vi "JSON Tree to MuxList.vi"(8 "error in (no error)":errorcluster, 11 "JSON Array":variant) -> (0 "error out":errorcluster, 2 "MuxList":cluster{"Src":string, "Dests":string[]}[](array[cluster]), 3 "JSON Tree Passthrough (JSON Array)":variant)   [LabVIEW 2015, in "SLSC Switch.lvlib" / "SLSC Switch.lvclass"]
uses:
  SLSC Switch.lvclass
  <vilib>/LVH/i3 JSON/JSON Parsing/Get Object Parameter Files/Get Object Parameter - Array.vi
  <vilib>/LVH/i3 JSON/JSON Parsing/Get Array Value at Index Files/Get Array Value at Index - Object.vi
  <vilib>/LVH/i3 JSON/JSON Parsing/Get Object Parameter Files/Get Object Parameter - String.vi
  <vilib>/LVH/i3 JSON/i3-json.lvlib
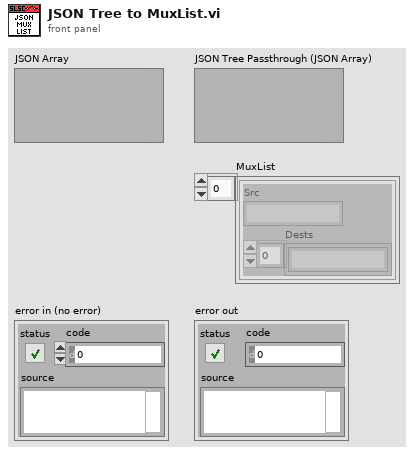
[diagram p1: front panel]
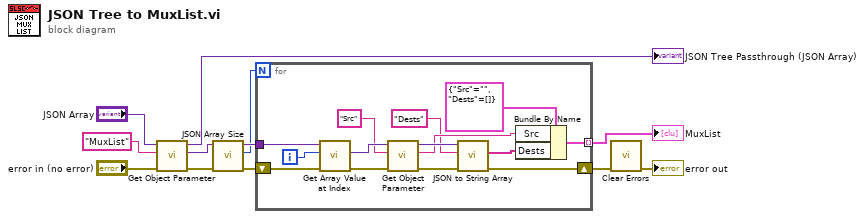
[diagram p0: block diagram]
diagram:
  n1 = call-poly <vilib>:"Get Object Parameter.vi"("error in (no error)"="error in (no error)", "Parameter Name"="MuxList", "JSON Tree In (JSON Object)"="JSON Array") -> ("error out"=w6:errorcluster, "JSON Array"=w5:variant, "JSON Tree Out Passthrough"=→"JSON Tree Passthrough (JSON Array)":variant)  [unwired: 5 in, 1 out]
  n2 = call <vilib>:"JSON Array Size.vi"("error in (no error)"=w6, "JSON Tree In (JSON Array)"=w5) -> ("error out"=w12:errorcluster, "Array Size"=w10:i32, "JSON Tree Passthrough (JSON Array)"=w11:variant)  [unwired: 7 in]
  n3 = for {
    N: w10 -> [_]
    tunnel: w11 -> [w26]
    tunnel: [w19] -> w3 mode=indexing
    shift-right: [w15] -> w2
    shift-left: w12 -> [w18]
    i -> [w25]
    n4 = call-poly <vilib>:"Get Array Value at Index.vi"("error in (no error)"=w18, "Index"=w25, "JSON Tree In (JSON Array)"=w26) -> ("error out"=w17:errorcluster, "JSON Object"=w24:variant)  [unwired: 5 in, 2 out]
    n5 = call-poly <vilib>:"Get Object Parameter.vi"("error in (no error)"=w17, "Parameter Name"="Src", "JSON Tree In (JSON Object)"=w24) -> ("error out"=w16:errorcluster, "String Value"=w21:string, "JSON Tree Out Passthrough"=w22:variant)  [unwired: 5 in, 1 out]
    n6 = call "JSON to String Array.vi"("error in (no error)"=w16, "Parameter Name"="Dests", "JSON Tree In"=w22) -> ("error out"=w15:errorcluster, "Array"=w14:string[])  [unwired: 6 in, 1 out]
    n7 = Bundle By Name(cluster=cluster{"Src":string, "Dests":string[]} {"Src"="", "Dests"=[]} ("MuxList"), "Src"=w21, "Dests"=w14) -> (w19:cluster{"Src":string, "Dests":string[]})
  }
  "MuxList" <- w3
  n8 = call <vilib>:"Clear Errors.vi"("error in (no error)"=w2) -> ("error out"=→"error out":errorcluster)  [unwired: 5 in, 1 out]
